vi "Measurement UI.vi"() -> ()   [LabVIEW 2021, in "Crosstalk_PMIC.lvlib"]
uses:
  Crosstalk_PMIC.lvlib
panel:
  in  "MeasGraphs":enum32{"Crosstalk", "Hidden Controls"}(tab)
  out "CrosstalkGraph":waveform(dbl)[](graph) caption="Ripple"
  out "Ripple values":dbl[](array[numeric])
  out "Max values":dbl[](array[numeric])
  out "Min values":dbl[](array[numeric])
  out "Load current":dbl
  out "Load voltage":dbl
  in  "Load resource name":string
  out "dt":dbl[](array[numeric])
  out "Scope amplitude":dbl[](array[numeric])
  in  "Scope channel names":string[](array[string])
  in  "Scope resource names":string[](array[string])
  in  "Source resource name":string caption="RESOURCE NAME"
  out "MeasTable":string[][](table)
  in  "ELOADResourceName":refnum<k15> caption="RESOURCE NAME"
  in  "ExportData":bool
  in  "Load current level":dbl=6.0 caption="CURRENT LEVEL" format="%#_6pA"
  in  "Scope probe attenuation":dbl=1.0 caption="PROBE ATTENUATION"
  in  "Scope acquisition time":dbl=3.0 caption="ACQUISTION TIME" format="%#_6ps"
  in  "Scope sample rate":dbl=10000.0 caption="SAMPLE RATE" format="%#_6pHz"
  in  "Scope channel parameters":T1(array[cluster]) caption="CHANNEL PARAMETERS"
  in  "Scope configuration":string="Scope configuration"
  out "Status":string
  in  "PPSResourceName":refnum<k15> caption="RESOURCE NAME"
  in  "DUT setup time":dbl=1.0 caption="DUT SETUP TIME" format="%#_6ps"
  in  "Source voltage level":dbl=12.0 caption="VOLTAGE LEVEL" format="%#_6pV"
  in  "Aperture time":dbl=0.005 caption="APERTURE TIME" format="%#_6ps"
  in  "Load voltage limit range":dbl=6.0 caption="VOLTAGE LIMIT RANGE" format="%#_6pV"
  in  "Source current limit":dbl=15.0 caption="CURRENT LIMIT" format="%#_6pA"
  in  "Load configuration":string="Load configuration"
  in  "Source configuration":string="Source configuration"
  in  "Measurement settings":string="Measurement settings"
  in  "Mode of operation":T2(ring)=enum."Perform measurement" caption="MODE OF OPERATION"
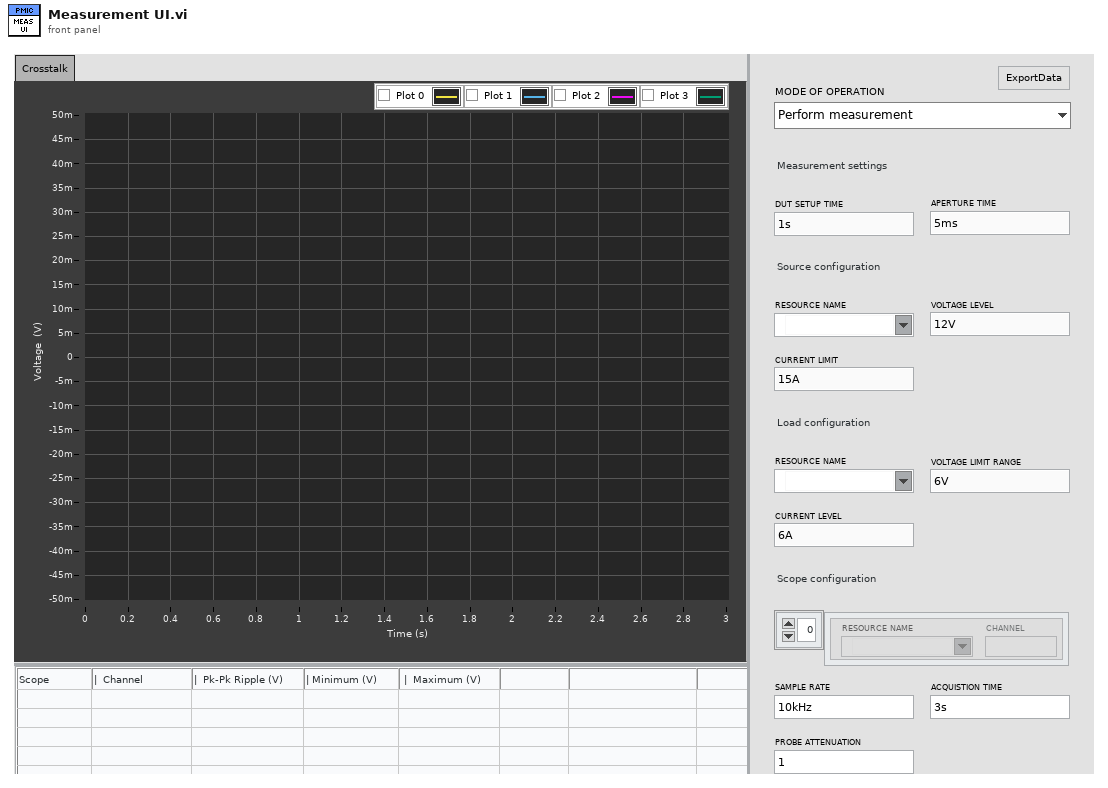
[diagram p1: front panel]
types:
  T1 = cluster{"ScopeResourceName":refnum<k15>, "Channel name":string}[]
  T2 = enum32{"Power on the DUT", "Perform measurement", "Power off the DUT"}
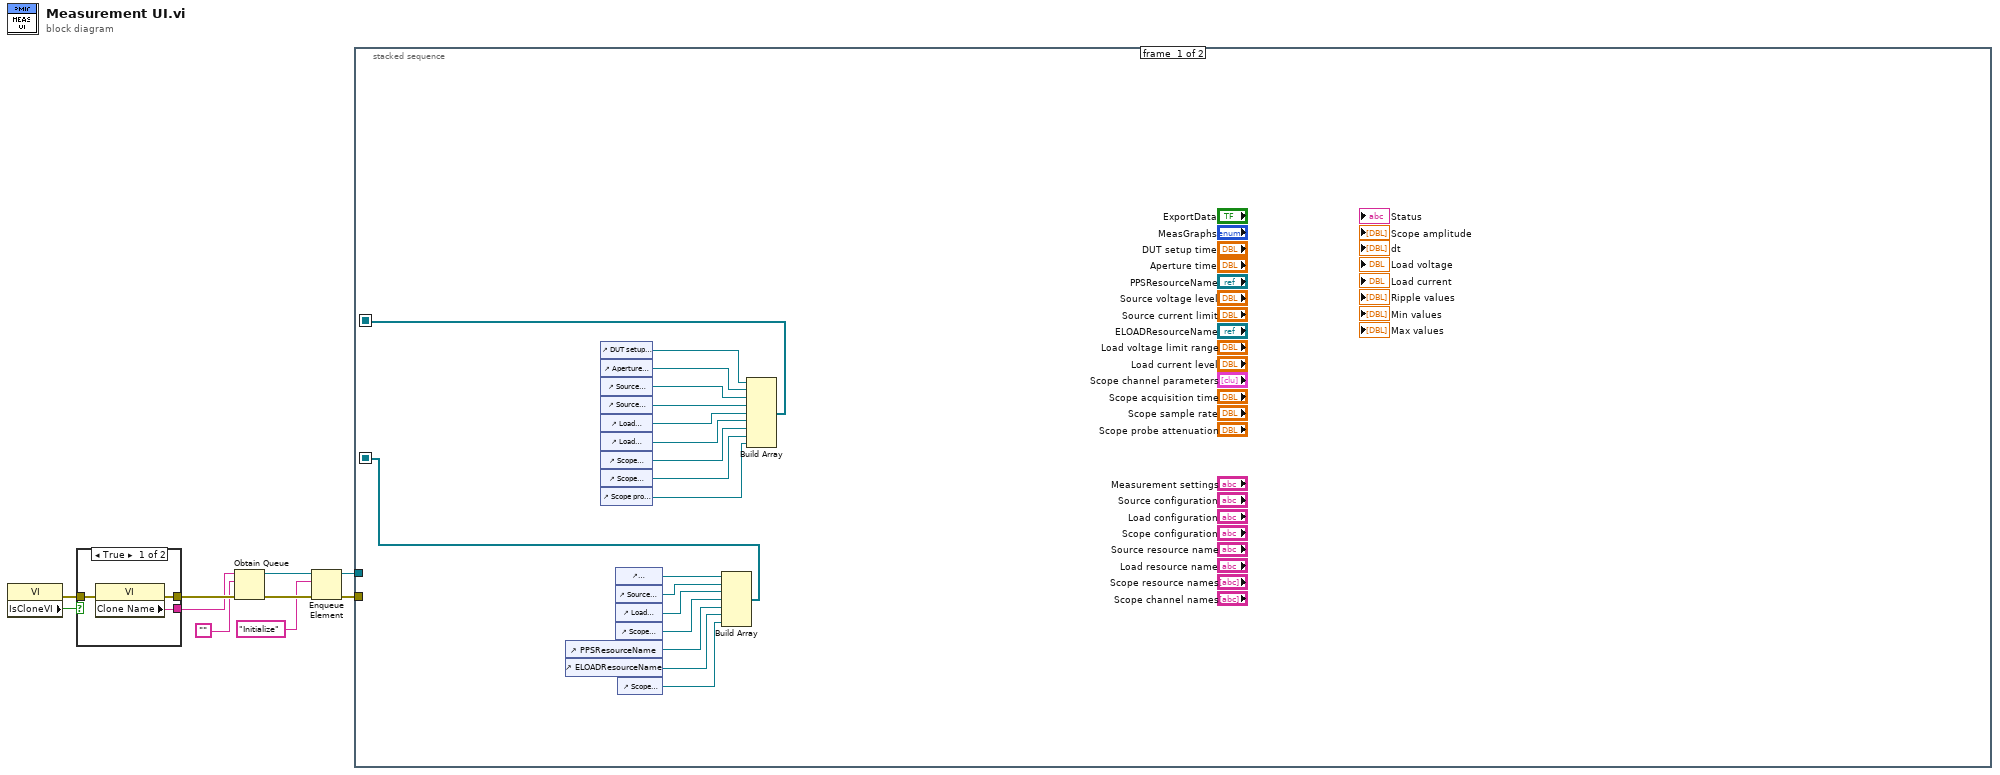
[diagram p0: block diagram]
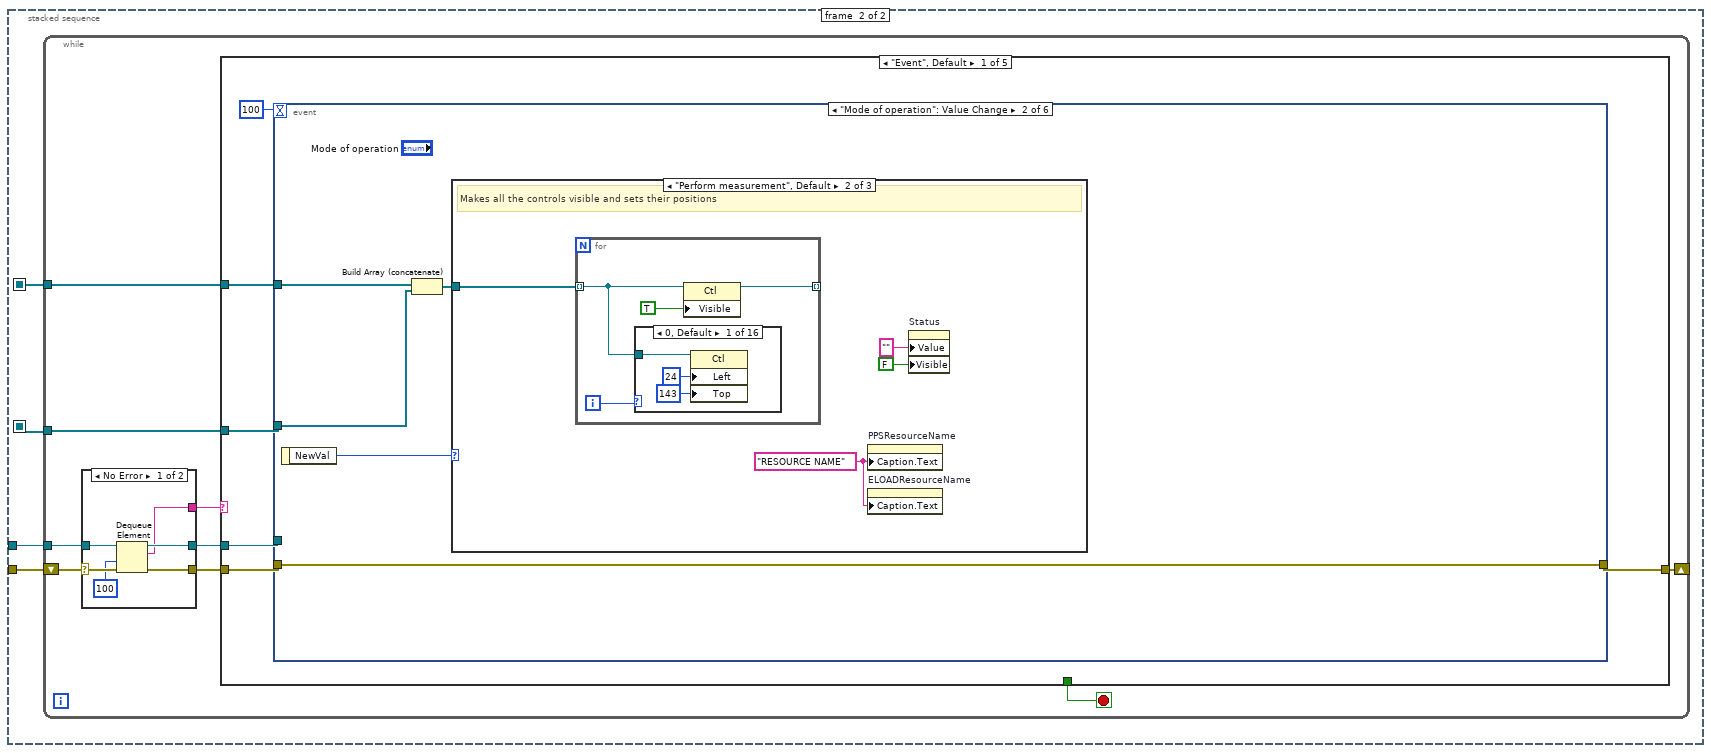
[diagram p2: hidden frame]
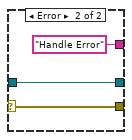
[diagram p3: hidden frame]
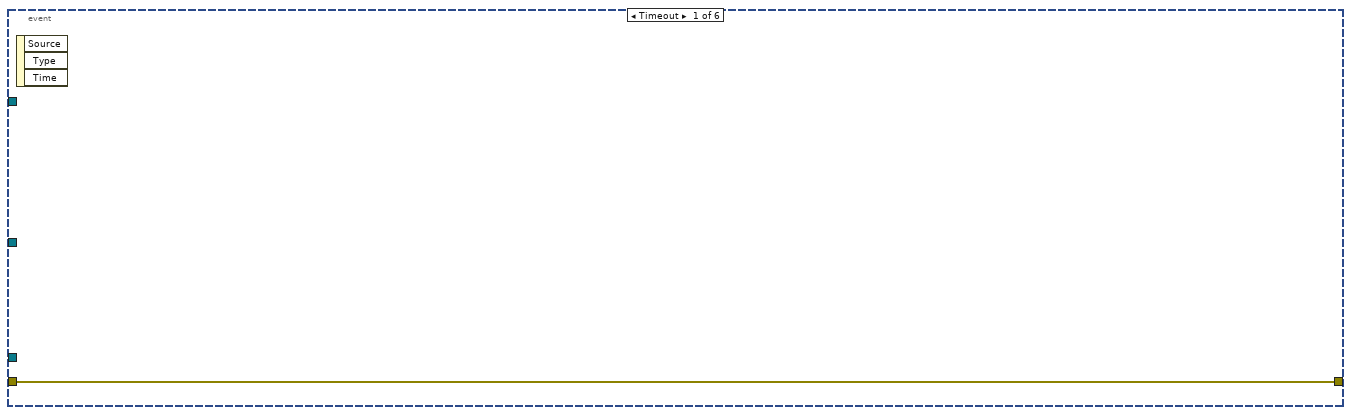
[diagram p4: hidden frame]
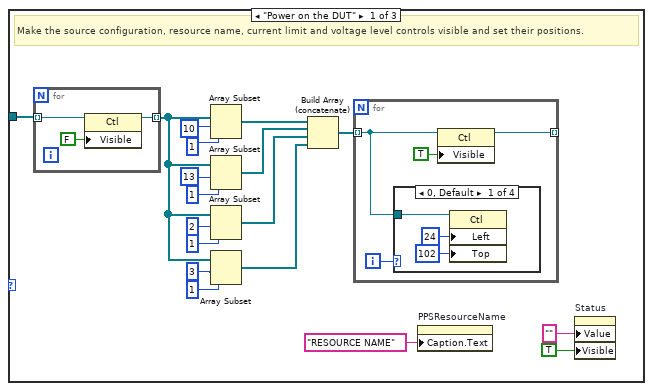
[diagram p5: hidden frame]
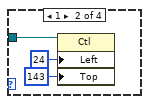
[diagram p6: hidden frame]
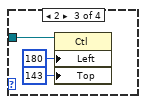
[diagram p7: hidden frame]
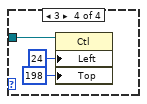
[diagram p8: hidden frame]
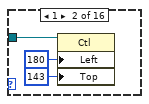
[diagram p9: hidden frame]
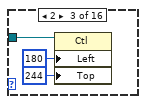
[diagram p10: hidden frame]
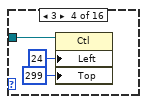
[diagram p11: hidden frame]
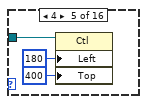
[diagram p12: hidden frame]
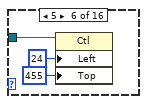
[diagram p13: hidden frame]
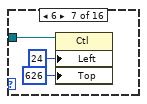
[diagram p14: hidden frame]
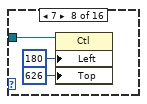
[diagram p15: hidden frame]
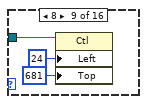
[diagram p16: hidden frame]
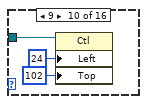
[diagram p17: hidden frame]
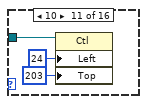
[diagram p18: hidden frame]
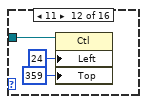
[diagram p19: hidden frame]
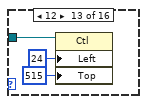
[diagram p20: hidden frame]
diagram:
  n1 = property class="VI"() -> (error out=w1:errorcluster, "IsCloneVI"=w2:bool)  [unwired: 2 in, 1 out]
  n2 = case shown="True" w2 {
    tunnel: [w13 w16] -> w10
    tunnel: [w12 w15] -> w9
    tunnel: w1 -> [w11 w14]
    frame True {
      n3 = property class="VI"(error in=w11) -> (error out=w13:errorcluster, "Clone Name"=w12:string)  [unwired: 1 in, 1 out]
    }
    frame False {
      n4 = property class="VI"(error in=w14) -> (error out=w16:errorcluster, "Name"=w15:string)  [unwired: 1 in, 1 out]
    }
  }
  n5 = Obtain Queue(name (unnamed)=w9, element data type="", error in (no error)=w10) -> (queue out=w6:refnum<queue>, error out=w8:errorcluster)  [unwired: 2 in, 1 out]
  n6 = Enqueue Element(queue=w6, element="Initialize", error in (no error)=w8) -> (queue out=w5:refnum<queue>, error out=w7:errorcluster)  [unwired: 1 in, 1 out]
  n7 = stacked-sequence {
    seq-local: [w28 _] -> [_ w36]
    seq-local: [w29 _] -> [_ w35]
    tunnel: w7 -> [_ w38]
    tunnel: w5 -> [_ w37]
    frame #0 {
      n8 = control-ref of="PPSResourceName"() -> (w31:refnum<vi>)
      n9 = control-ref of="ELOADResourceName"() -> (w30:refnum<vi>)
      n10 = control-ref of="DUT setup time"() -> (w27:refnum<vi>)
      n11 = control-ref of="Aperture time"() -> (w26:refnum<vi>)
      n12 = control-ref of="Source voltage level"() -> (w25:refnum<vi>)
      n13 = control-ref of="Source current limit"() -> (w24:refnum<vi>)
      n14 = control-ref of="Load voltage limit range"() -> (w23:refnum<vi>)
      n15 = control-ref of="Load current level"() -> (w22:refnum<vi>)
      n16 = control-ref of="Scope sample rate"() -> (w21:refnum<vi>)
      n17 = control-ref of="Scope acquisition time"() -> (w20:refnum<vi>)
      n18 = control-ref of="Scope probe attenuation"() -> (w19:refnum<vi>)
      n19 = control-ref of="Measurement settings"() -> (w34:refnum<vi>)
      n20 = control-ref of="Source configuration"() -> (w32:refnum<vi>)
      n21 = control-ref of="Load configuration"() -> (w33:refnum<vi>)
      n22 = control-ref of="Scope configuration"() -> (w17:refnum<vi>)
      n23 = control-ref of="Scope channel parameters"() -> (w18:refnum<vi>)
      n24 = Build Array(w34, w32, w33, w17, w31, w30, w18) -> (w29:refnum<vi>[])
      n25 = Build Array(w27, w26, w25, w24, w23, w22, w21, w20, w19) -> (w28:refnum<vi>[])
    }
    frame #1 {
      n26 = while {
        shift-right: [w42] -> _
        shift-left: w38 -> [w47]
        tunnel: w37 -> [w45]
        tunnel: w36 -> [w40]
        tunnel: w35 -> [w39]
        stop <- w41 stop-if-true
        n27 = case shown="No Error" w47 {
          selector: w47 -> [w53 w56]
          tunnel: [w52 w56] -> w46
          tunnel: w45 -> [w51 w55]
          tunnel: [w50 w55] -> w44
          tunnel: [w49 "Handle Error"] -> w43
          frame No Error {
            n28 = Dequeue Element(queue=w51, timeout in ms (-1)=100, error in (no error)=w53) -> (queue out=w50:refnum<queue>, element=w49:string, error out=w52:errorcluster)  [unwired: 1 out]
          }
          frame Error {
          }
        }
        n29 = case shown="\"Event\", Default" w43 {
          tunnel: w46 -> [w61 w202 w217 w263 w264]
          tunnel: w44 -> [w59 _ _ w261 _]
          tunnel: [w62 w202 w217 w255 w264] -> w42
          tunnel: [_ _ _ TRUE _] -> w41
          tunnel: w40 -> [w58 _ _ w254 _]
          tunnel: w39 -> [w57 _ _ w253 _]
          frame "Event", Default {
            n30 = event shown="[1] \"Mode of operation\": Value Change" {
              selector: _ -> [_ _ _ _ _ _]
              dyn-events: _ -> [_ _ _ _ _ _]
              timeout: 100 -> [_ _ _ _ _ _]
              tunnel: [w63 w64 w184 w187 _ w196] -> w62
              tunnel: w61 -> [w63 w64 w184 w187 _ w197]
              tunnel: w59 -> [_ _ _ _ _ w195]
              tunnel: w58 -> [_ w65 _ _ _ _]
              tunnel: w57 -> [_ w67 _ _ _ _]
              event Timeout {
                n31 = event-data() -> ()  [unwired: 1 in, 3 out]
              }
              event "Mode of operation": Value Change {
                n32 = event-data() -> ("NewVal"=w68:T2)  [unwired: 1 in]
                n33 = Build Array (concatenate)(w65, w67) -> (w66:refnum<vi>[])
                n34 = case shown="\"Perform measurement\", Default" w68 {
                  tunnel: w66 -> [w78 w109 w167]
                  frame "Power on the DUT" {
                    # "Make the source configuration, resource name, current limit and voltage level controls visible and set their positions."
                    n35 = for {
                      tunnel: w78 -> [w89] mode=indexing
                      tunnel: [w87] -> w75 mode=indexing
                      n36 = property class="Ctl"(reference=w89, "Visible"=FALSE) -> (reference out=w87:refnum<vi>)  [unwired: 1 in, 1 out]
                    }
                    n37 = Array Subset(array=w75, index=10 ("length"), length=1 ("index")) -> (w77:refnum<vi>[])
                    n38 = Array Subset(array=w75, index=13 ("length"), length=1 ("index")) -> (w76:refnum<vi>[])
                    n39 = Array Subset(array=w75, index=2 ("length"), length=1 ("index")) -> (w74:refnum<vi>[])
                    n40 = Array Subset(array=w75, index=3 ("length"), length=1 ("index")) -> (w72:refnum<vi>[])
                    n41 = Build Array (concatenate)(w77, w76, w74, w72) -> (w73:refnum<vi>[])
                    n42 = for {
                      tunnel: [w92] -> _ mode=indexing
                      tunnel: w73 -> [w90] mode=indexing
                      i -> [w91]
                      n43 = case shown="0, Default" w91 {
                        tunnel: w90 -> [w96 w99 w102 w105]
                        frame 0, Default {
                          n44 = property class="Ctl"(reference=w96, "Left"=24 ("Position:Left"), "Top"=102 ("Position:Top")) -> ()  [unwired: 1 in, 2 out]
                        }
                        frame 1 {
                          n45 = property class="Ctl"(reference=w99, "Left"=24 ("Position:Left"), "Top"=143 ("Position:Top")) -> ()  [unwired: 1 in, 2 out]
                        }
                        frame 2 {
                          n46 = property class="Ctl"(reference=w102, "Left"=180 ("Position:Left"), "Top"=143 ("Position:Top")) -> ()  [unwired: 1 in, 2 out]
                        }
                        frame 3 {
                          n47 = property class="Ctl"(reference=w105, "Left"=24 ("Position:Left"), "Top"=198 ("Position:Top")) -> ()  [unwired: 1 in, 2 out]
                        }
                      }
                      n48 = property class="Ctl"(reference=w90, "Visible"=TRUE) -> (reference out=w92:refnum<vi>)  [unwired: 1 in, 1 out]
                    }
                    n49 = property on="PPSResourceName" class="IVIName"("Caption.Text"="RESOURCE NAME") -> ()  [unwired: 2 in, 2 out]
                    n50 = property on="Status" class="Str"("Value"="" ("Status"), "Visible"=TRUE) -> ()  [unwired: 2 in, 2 out]
                  }
                  frame "Perform measurement", Default {
                    w108 = "RESOURCE NAME" ("Caption.Text")
                    # "Makes all the controls visible and sets their positions"
                    n51 = for {
                      tunnel: w109 -> [w110] mode=indexing
                      tunnel: [w112] -> _ mode=indexing
                      i -> [w111]
                      n52 = case shown="0, Default" w111 {
                        tunnel: w110 -> [w116 w119 w122 w125 w128 w131 w134 w137 w140 w143 w146 w149 w152 w155 w158 w161]
                        frame 0, Default {
                          n53 = property class="Ctl"(reference=w116, "Left"=24 ("Position:Left"), "Top"=143 ("Position:Top")) -> ()  [unwired: 1 in, 2 out]
                        }
                        frame 1 {
                          n54 = property class="Ctl"(reference=w119, "Left"=180 ("Position:Left"), "Top"=143 ("Position:Top")) -> ()  [unwired: 1 in, 2 out]
                        }
                        frame 2 {
                          n55 = property class="Ctl"(reference=w122, "Left"=180 ("Position:Left"), "Top"=244 ("Position:Top")) -> ()  [unwired: 1 in, 2 out]
                        }
                        frame 3 {
                          n56 = property class="Ctl"(reference=w125, "Left"=24 ("Position:Left"), "Top"=299 ("Position:Top")) -> ()  [unwired: 1 in, 2 out]
                        }
                        frame 4 {
                          n57 = property class="Ctl"(reference=w128, "Left"=180 ("Position:Left"), "Top"=400 ("Position:Top")) -> ()  [unwired: 1 in, 2 out]
                        }
                        frame 5 {
                          n58 = property class="Ctl"(reference=w131, "Left"=24 ("Position:Left"), "Top"=455 ("Position:Top")) -> ()  [unwired: 1 in, 2 out]
                        }
                        frame 6 {
                          n59 = property class="Ctl"(reference=w134, "Left"=24 ("Position:Left"), "Top"=626 ("Position:Top")) -> ()  [unwired: 1 in, 2 out]
                        }
                        frame 7 {
                          n60 = property class="Ctl"(reference=w137, "Left"=180 ("Position:Left"), "Top"=626 ("Position:Top")) -> ()  [unwired: 1 in, 2 out]
                        }
                        frame 8 {
                          n61 = property class="Ctl"(reference=w140, "Left"=24 ("Position:Left"), "Top"=681 ("Position:Top")) -> ()  [unwired: 1 in, 2 out]
                        }
                        frame 9 {
                          n62 = property class="Ctl"(reference=w143, "Left"=24 ("Position:Left"), "Top"=102 ("Position:Top")) -> ()  [unwired: 1 in, 2 out]
                        }
                        frame 10 {
                          n63 = property class="Ctl"(reference=w146, "Left"=24 ("Position:Left"), "Top"=203 ("Position:Top")) -> ()  [unwired: 1 in, 2 out]
                        }
                        frame 11 {
                          n64 = property class="Ctl"(reference=w149, "Left"=24 ("Position:Left"), "Top"=359 ("Position:Top")) -> ()  [unwired: 1 in, 2 out]
                        }
                        frame 12 {
                          n65 = property class="Ctl"(reference=w152, "Left"=24 ("Position:Left"), "Top"=515 ("Position:Top")) -> ()  [unwired: 1 in, 2 out]
                        }
                        frame 13 {
                          n66 = property class="Ctl"(reference=w155, "Left"=24 ("Position:Left"), "Top"=244 ("Position:Top")) -> ()  [unwired: 1 in, 2 out]
                        }
                        frame 14 {
                          n67 = property class="Ctl"(reference=w158, "Left"=24 ("Position:Left"), "Top"=400 ("Position:Top")) -> ()  [unwired: 1 in, 2 out]
                        }
                        frame 15 {
                          n68 = property class="Ctl"(reference=w161, "Left"=24 ("Position:Left"), "Top"=556 ("Position:Top")) -> ()  [unwired: 1 in, 2 out]
                        }
                      }
                      n69 = property class="Ctl"(reference=w110, "Visible"=TRUE) -> (reference out=w112:refnum<vi>)  [unwired: 1 in, 1 out]
                    }
                    n70 = property on="PPSResourceName" class="IVIName"("Caption.Text"=w108) -> ()  [unwired: 2 in, 2 out]
                    n71 = property on="ELOADResourceName" class="IVIName"("Caption.Text"=w108) -> ()  [unwired: 2 in, 2 out]
                    n72 = property on="Status" class="Str"("Value"="" ("Status"), "Visible"=FALSE) -> ()  [unwired: 2 in, 2 out]
                  }
                  frame "Power off the DUT" {
                    # "Makes only the Source and Load Resource Name controls visible and sets their positions"
                    n73 = for {
                      tunnel: w167 -> [w172] mode=indexing
                      tunnel: [w171] -> w166 mode=indexing
                      n74 = property class="Ctl"(reference=w172, "Visible"=FALSE) -> (reference out=w171:refnum<vi>)  [unwired: 1 in, 1 out]
                    }
                    n75 = Array Subset(array=w166, index=13 ("length"), length=2 ("index")) -> (w168:refnum<vi>[])
                    n76 = property on="PPSResourceName" class="IVIName"("Caption.Text"="SOURCE RESOURCE NAME") -> ()  [unwired: 2 in, 2 out]
                    n77 = property on="ELOADResourceName" class="IVIName"("Caption.Text"="LOAD RESOURCE NAME") -> ()  [unwired: 2 in, 2 out]
                    n78 = for {
                      tunnel: w168 -> [w174] mode=indexing
                      tunnel: [w176] -> _ mode=indexing
                      i -> [w175]
                      n79 = case shown="0, Default" w175 {
                        tunnel: w174 -> [w180 w183]
                        frame 0, Default {
                          n80 = property class="Ctl"(reference=w180, "Left"=24 ("Position:Left"), "Top"=102 ("Position:Top")) -> ()  [unwired: 1 in, 2 out]
                        }
                        frame 1 {
                          n81 = property class="Ctl"(reference=w183, "Left"=24 ("Position:Left"), "Top"=157 ("Position:Top")) -> ()  [unwired: 1 in, 2 out]
                        }
                      }
                      n82 = property class="Ctl"(reference=w174, "Visible"=TRUE) -> (reference out=w176:refnum<vi>)  [unwired: 1 in, 1 out]
                    }
                    n83 = property on="Status" class="Str"("Value"="" ("Status"), "Visible"=TRUE) -> ()  [unwired: 2 in, 2 out]
                  }
                }
              }
              event "PPSResourceName": Value Change {
                n84 = event-data() -> ()  [unwired: 1 in, 1 out]
                n85 = property on="PPSResourceName" class="IVIName"() -> ("Value"=w185:refnum<k15>)  [unwired: 2 in, 2 out]
                n86 = property on="Source resource name" class="Str"("Value"=w185) -> ()  [unwired: 2 in, 2 out]
              }
              event "ELOADResourceName": Value Change {
                n87 = event-data() -> ("NewVal"=w186:refnum<k15>)  [unwired: 1 in]
                n88 = property on="Load resource name" class="Str"("Value"=w186) -> ()  [unwired: 2 in, 2 out]
              }
              event "Scope channel parameters": Value Change {
                n89 = event-data() -> ("NewVal"=w190:T1)  [unwired: 1 in]
                n90 = for {
                  tunnel: w190 -> [w193] mode=indexing
                  tunnel: [w192] -> w189 mode=indexing
                  tunnel: [w191] -> w188 mode=indexing
                  n91 = Unbundle By Name(w193) -> ("ScopeResourceName"=w192:refnum<k15>, "Channel name"=w191:string)
                }
                n92 = property on="Scope channel names" class="Arr (strict)"("Value"=w188) -> ()  [unwired: 2 in, 2 out]
                n93 = property on="Scope resource names" class="Arr (strict)"("Value"=w189) -> ()  [unwired: 2 in, 2 out]
              }
              event Panel Close? {
                n94 = event-data() -> ()  [unwired: 1 in, 4 out]
                n95 = Enqueue Element(queue=w195, element="Exit", error in (no error)=w197) -> (error out=w196:errorcluster)  [unwired: 1 in, 2 out]
                n96 = event-data("Discard?"=TRUE) -> ()  [unwired: 1 in, 1 out]
              }
            }
          }
          frame "Initialize" {
            w201 = "<Select Device>"
            n97 = property on="PPSResourceName" class="IVIName"("Value"=w201) -> ()  [unwired: 2 in, 2 out]
            n98 = property on="ELOADResourceName" class="IVIName"("Value"=w201) -> ()  [unwired: 2 in, 2 out]
            n99 = property on="Status" class="Str"("Visible"=FALSE) -> ()  [unwired: 2 in, 2 out]
            n100 = property on="CrosstalkGraph" class="WFGraph (strict)"("ActPaletteTool"=2 ("Palette:Active Tool")) -> ()  [unwired: 2 in, 2 out]
          }
          frame "Post UI Update" {
            # "This case will be triggered, after framework updates the User interface with result values."
            n101 = local read "Scope amplitude"() -> (w215:dbl[])
            n102 = local read "dt"() -> (w214:dbl[])
            n103 = property on="Scope channel parameters" class="Arr (strict)"() -> ("Value"=w205:T1)  [unwired: 2 in, 2 out]
            n104 = Array Size(array=w215) -> (size(s)=w212:i32)
            n105 = Array Size(array=w214) -> (size(s)=w213:i32)
            n106 = Divide(x=w212, y=w213) -> (x/y=w211:dbl)
            n107 = for {
              tunnel: w205 -> [w226] mode=indexing
              tunnel: [w221] -> w206 mode=concatenating
              tunnel: [w218] -> w204 mode=concatenating
              n108 = Unbundle By Name(w226) -> ("ScopeResourceName"=w219:refnum<k15>, "Channel name"=w222:string)
              n109 = Spreadsheet String To Array(delimiter (Tab)=",", format string="%s", spreadsheet string=w222, array type (2D Dbl)=string[] []) -> (array=w221:string[])
              n110 = Array Size(array=w221) -> (size(s)=w220:i32)
              n111 = for {
                N: w220 -> [_]
                tunnel: w219 -> [w227]
                tunnel: [w227] -> w218 mode=indexing
              }
            }
            n112 = for {
              tunnel: [w251] -> w216 mode=indexing
              tunnel: w214 -> [w250] mode=indexing
              shift-right: [w248] -> _
              shift-left: w215 -> [w249]
              tunnel: w211 -> [w247]
              n113 = Delete From Array(array=w249, length=w247, index=0) -> (deleted portion=w245:dbl[], array with subset deleted=w248:dbl[])
              n114 = Bundle By Name("Y"=w245, "dt"=w250) -> (w251:waveform(dbl))  [unwired: 1 in]
            }
            "CrosstalkGraph" <- w216
            n115 = local write "ExportData"(FALSE ("ExportData")) -> ()
            n116 = local read "Ripple values"() -> (w209:dbl[])
            n117 = local read "Max values"() -> (w207:dbl[])
            n118 = local read "Min values"() -> (w208:dbl[])
            n119 = for {
              tunnel: [w235] -> w210 mode=indexing
              tunnel: w209 -> [w239] mode=indexing
              tunnel: w208 -> [w238] mode=indexing
              tunnel: w207 -> [w237] mode=indexing
              tunnel: w206 -> [w232] mode=indexing
              tunnel: w204 -> [w234] mode=indexing
              w230 = "|   " ("initial string")
              n120 = Format Into String(format string="%s", w234) -> (resulting string=w228:string)  [unwired: 2 in, 1 out]
              n121 = Format Into String(format string="%s", initial string=w230, w232) -> (resulting string=w233:string)  [unwired: 1 in, 1 out]
              n122 = Format Into String(format string="%.6f" ("initial string"), initial string=w230, w239) -> (resulting string=w241:string)  [unwired: 1 in, 1 out]
              n123 = Format Into String(format string="%.6f" ("initial string"), initial string=w230, w238) -> (resulting string=w242:string)  [unwired: 1 in, 1 out]
              n124 = Format Into String(format string="%.6f" ("initial string"), initial string=w230, w237) -> (resulting string=w236:string)  [unwired: 1 in, 1 out]
              n125 = Build Array(w228, w233, w241, w242, w236) -> (w235:string[])
            }
            "MeasTable" <- w210
          }
          frame "Exit" {
            # "This case is triggered to close the User Interface from framework"
            n126 = Build Array (concatenate)(w254, w253) -> (w252:refnum<vi>[])
            n127 = Close Reference(reference=w252) -> (error out=w257:errorcluster)  [unwired: 1 in]
            n128 = Flush Queue(queue=w261, error in (no error)=w263) -> (queue out=w260:refnum<queue>, error out=w259:errorcluster)  [unwired: 1 out]
            n129 = Release Queue(queue=w260, force destroy? (F)=TRUE, error in (no error)=w259) -> (error out=w256:errorcluster)  [unwired: 2 out]
            n130 = Merge Errors(w257, w256) -> (w255:errorcluster)
          }
          frame "Handle Error" {
          }
        }
      }
    }
  }
